vi "StartCapture.vi"(8 "error in (no error)":errorcluster, 10 "Continuous":bool, 11 "Hamamatsu_Camera in":refnum<class "Hamamatsu_Camera.lvclass">) -> (0 "error out":errorcluster, 3 "Hamamatsu_Camera out":refnum<class "Hamamatsu_Camera.lvclass">)   [LabVIEW 2023, in "CameraLibrary.lvlib" / "Hamamatsu_Camera.lvlib" / "Hamamatsu_Camera.lvclass"]
uses:
  Hamamatsu_Camera.lvclass
  C:/Program Files/National Instruments/LabVIEW 2023/vi.lib/ActorFramework/Actor/Actor.lvclass
  Hamamatsu_Camera.lvclass/Hamamatsu_Camera.ctl
  <vilib>/ActorFramework/Actor/Actor.lvclass/Actor.ctl
  <vilib>/ActorFramework/Message Enqueuer/Message Enqueuer.lvclass/Message Enqueuer.ctl
  <vilib>/ActorFramework/Message Enqueuer/Enqueue.vi
  Interfaces/AbstractInstrumentClasses/Cameras_LV/CameraComm Messages/Capture Started Msg/Capture Started Msg.lvclass
  C:/Program Files/National Instruments/LabVIEW 2023/vi.lib/ActorFramework/Message/Message.lvclass
  <vilib>/ActorFramework/Message Priority Queue/Priority Enqueue.vi
  <vilib>/ActorFramework/Actor/Actor.lvclass
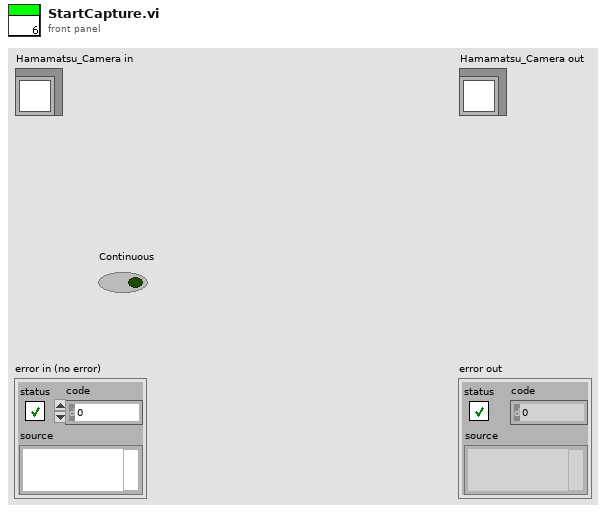
[diagram p1: front panel]
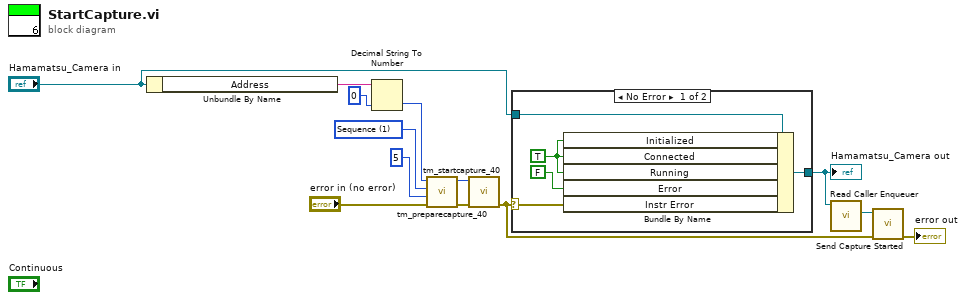
[diagram p0: block diagram]
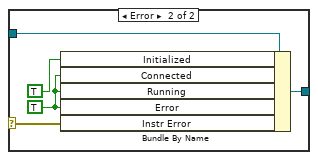
[diagram p2: hidden frame]
diagram:
  w5 = 1 items=["Snap", "Sequence"] ("Capture mode")
  n1 = Unbundle By Name("Hamamatsu_Camera in") -> ("Address"=w13:string)
  n2 = Decimal String To Number(string=w13, default (0L)=u32 0 ("default (0 I32)")) -> (number=w8:u32)  [unwired: 1 in, 1 out]
  n3 = call "tm_preparecapture_40.vi"("error in (no error)"="error in (no error)", "Frames"=5, "Capture mode"=w5, "Handle in"=w8) -> ("error out"=w6:errorcluster, "Handle out"=w9:u32)  [unwired: 4 in, 2 out]
  n4 = call "tm_startcapture_40.vi"("error in (no error)"=w6, "Handle in"=w9) -> ("error out"=w3:errorcluster)  [unwired: 8 in, 1 out]
  n5 = case shown="No Error" w3 {
    selector: w3 -> [w15 w20]
    tunnel: "Hamamatsu_Camera in" -> [w18 w23]
    tunnel: [w16 w21] -> w2
    frame No Error {
      w14 = TRUE ("InstrumentData.CurrentState.Connected")
      n6 = Bundle By Name(cluster=w18, "Initialized"=w14, "Connected"=w14, "Running"=w14, "Error"=FALSE ("InstrumentData.CurrentState.Initialized"), "Instr Error"=w15) -> (w16:refnum<class "Hamamatsu_Camera.lvclass">)
    }
    frame Error {
      w19 = TRUE ("InstrumentData.CurrentState.Connected")
      n7 = Bundle By Name(cluster=w23, "Initialized"=TRUE ("InstrumentData.CurrentState.Initialized"), "Connected"=w19, "Running"=w19, "Error"=w19, "Instr Error"=w20) -> (w21:refnum<class "Hamamatsu_Camera.lvclass">)
    }
  }
  "Hamamatsu_Camera out" <- w2
  n8 = call <vilib>:"Read Caller Enqueuer.vi"("Actor"=w2) -> ("Caller Enqueuer"=w11:refnum<class "Message Enqueuer.lvclass">)  [unwired: 10 in]
  n9 = call "Send Capture Started.vi"("error in (no error)"=w3, "Message Enqueuer"=w11) -> ("error out"=→"error out":errorcluster)  [unwired: 8 in, 1 out]
